vi "esp301 calculate timeout.vi"(9 "Arg":string, 10 "Velocity (units/s)":dbl, 11 "Position (units)":dbl) -> (2 "Numeric":dbl, 3 "Numeric 2":dbl)   [LabVIEW 2020, in "ESP301.lvclass"]
uses:
  ESP301.lvclass
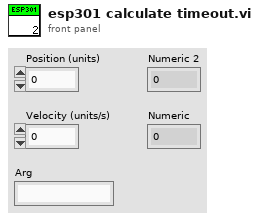
[diagram p1: front panel]
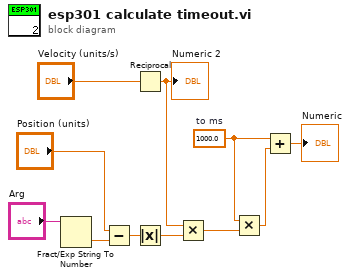
[diagram p0: block diagram]
diagram:
  w3 = 1000.0  # to ms
  n1 = Fract/Exp String To Number(string="Arg") -> (number=w4:dbl)  [unwired: 3 in, 1 out]
  n2 = Subtract(x="Position (units)", y=w4) -> (x-y=w5:dbl)
  n3 = Reciprocal(x="Velocity (units/s)") -> (1/x=w7:dbl)
  "Numeric 2" <- w7
  n4 = Absolute Value(x=w5) -> (abs(x)=w6:dbl)
  n5 = Multiply(x=w7, y=w6) -> (x*y=w1:dbl)
  n6 = Multiply(x=w3, y=w1) -> (x*y=w2:dbl)
  n7 = Add(x=w3, y=w2) -> (x+y=→"Numeric":dbl)
